vi "Read Nested Actor.vi"(11 "Caller Endpoint in":refnum<class "Caller Endpoint.lvclass">) -> (2 "Nested Actor":refnum<class "Actor.lvclass">)   [LabVIEW 2020, in "Caller Endpoint.lvlib" / "Caller Endpoint.lvclass"]
doc: "Use this read accessor to obtain an instance of the actor launched by the Caller Endpoint."
uses:
  Caller Endpoint.lvclass
  <vilib>/ActorFramework/Actor/Actor.lvclass
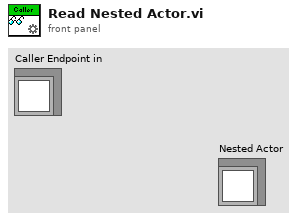
[diagram p1: front panel]
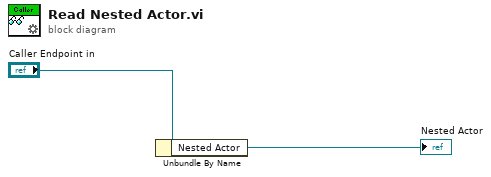
[diagram p0: block diagram]
diagram:
  n1 = Unbundle By Name("Caller Endpoint in") -> ("Nested Actor"=→"Nested Actor":refnum<class "Actor.lvclass">)
